vi "SimulatedContinuous.vi"(8 "error in (no error)":errorcluster, 11 "first block":bool) -> (0 "error out":errorcluster, 3 "signal out":waveform(dbl), 5 "Channel":string)   [LabVIEW 2017, in "EmsaAcquisition.lvlib"]
uses:
  <vilib>/addons/InsightCM/Devices/Shared/Emsa/EmsaAcquisition/EmsaAcquisition.lvlib
  <vilib>/addons/InsightCM/Devices/Shared/Emsa/EmsaAcquisition/subVIs/SimulatedConfigRefGlobal.vi
  <vilib>/measure/NI_MABase.lvlib
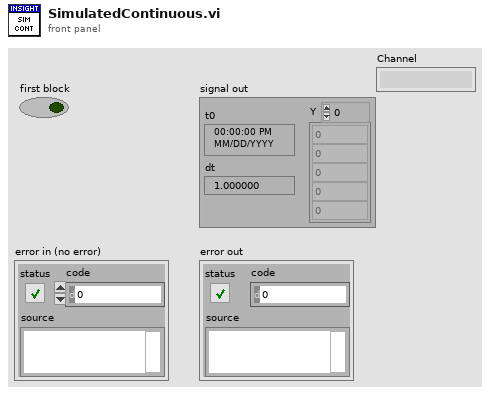
[diagram p1: front panel]
types:
  T1 = typedef "EmsaAcquisition.lvlib/SimulatedConfigRefs.ctl" = cluster{"SimulatedSignalConfig":refnum<vi>}
  T2 = typedef "EmsaAcquisition.lvlib/SimulatedSignalConfig.ctl" = cluster{"Channel Name":string[], "Valid":bool[], "Hardware Channel":string[], "Unit":string[], "Sweep Configs":T3[]}
  T3 = typedef "EmsaAcquisition.lvlib/SimulatedSweepConfig.ctl" = cluster{"Sweep Frequency List":cluster{"frequency":dbl, "bandwidth":dbl}[], "Detection Time":dbl, "Detection Mode":enum16{"Peak", "Quasi Peak", "Average"}, "Full Scale Volts":dbl, "Total Sweep Pts":i32, "Sweep Pointer":i32, "Sweep":T4[], "Sweep Start Time":timestamp}
  T4 = typedef "EmsaAcquisition.lvlib/SweepElement.ctl" = cluster{"Frequency":dbl, "Amplitude":dbl}
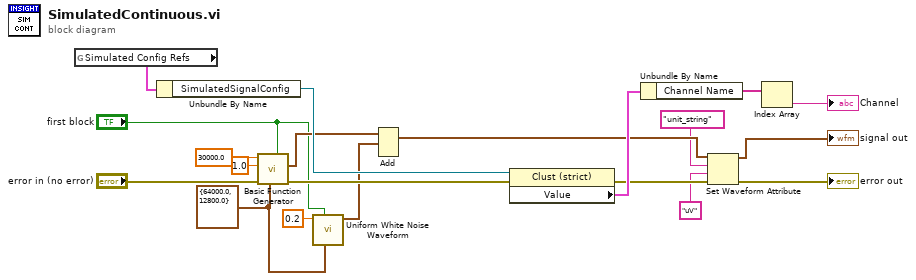
[diagram p0: block diagram]
diagram:
  w10 = cluster{"Fs":dbl, "#s":dbl} {"Fs"=64000.0, "#s"=12800.0} ("sampling info")
  n1 = global read "SimulatedConfigRefGlobal.vi" "Simulated Config Refs"() -> (w18:T1)
  n2 = Unbundle By Name(w18) -> ("SimulatedSignalConfig"=w17:refnum<vi>)
  n3 = call <vilib>:"Basic Function Generator.vi"("reset signal"="first block", "sampling info"=w10, "error in (no error)"="error in (no error)", "amplitude"=1.0, "frequency"=30000.0) -> ("error out"=w15:errorcluster, "signal out"=w12:waveform(dbl))  [unwired: 4 in, 1 out]
  n4 = call <vilib>:"Uniform White Noise Waveform.vi"("sampling info"=w10, "reset signal"="first block", "amplitude"=0.2) -> ("signal out"=w11:waveform(dbl))  [unwired: 7 in, 1 out]
  n5 = Add(1:w11, 2:w12) -> (0:w4:waveform(dbl))  [unwired: 1 in, 1 out]
  n6 = property class="Clust (strict)"(reference=w17, error in=w15) -> (error out=w6:errorcluster, "Value"=w16:T2)  [unwired: 1 out]
  n7 = Unbundle By Name(w16) -> ("Channel Name"=w14:string[])
  n8 = Set Waveform Attribute(4:w6, 5:"uV" ("name"), 6:"unit_string" ("name"), 7:w4) -> (0:→"error out":errorcluster, 3:→"signal out":waveform(dbl))  [unwired: 1 out]
  n9 = Index Array(array=w14) -> (element=→"Channel":string)  [unwired: 1 in]
